vi "test Verify a VI.vi"(8 "error in":errorcluster, 11 "Test Case In":refnum<class "LUnit Extensions Tests.lvclass">) -> (0 "error out":errorcluster, 3 "Test Case Out":refnum<class "LUnit Extensions Tests.lvclass">)   [LabVIEW 2020, in "LUnit Extensions Tests.lvclass"]
uses:
  LUnit Extensions Tests.lvclass
  C:/Program Files/National Instruments/LabVIEW 2026/vi.lib/Astemes/LUnit/Test Case.lvclass
  Source/Extensions/LUnit.Extension/LUnit.Extension.lvlib
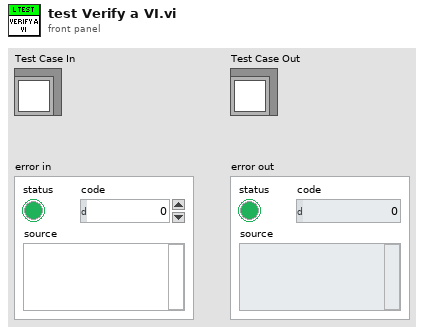
[diagram p1: front panel]
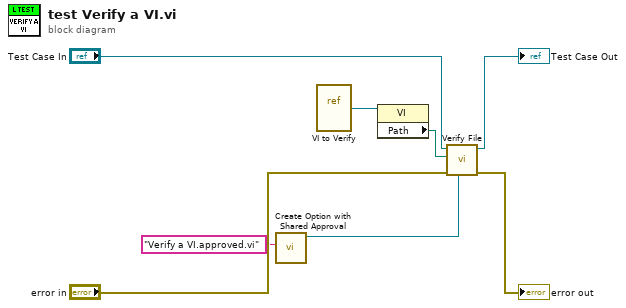
[diagram p0: block diagram]
diagram:
  n1 = call "Create Option with Shared Approval.vi"("Filename"="Verify a VI.approved.vi") -> ("Options outs"=w2:refnum<class "Options.lvclass">)  [unwired: 10 in]
  n2 = vi-ref "VI to Verify.vi"() -> (w4:refnum<vi>)
  n3 = property class="VI"(reference=w4) -> ("Path"=w3:path)  [unwired: 1 in, 2 out]
  n4 = call "Verify File.vi"("Options"=w2, "error in"="error in", "path to file"=w3, "LUnit Test Case In"="Test Case In") -> ("error out"=→"error out":errorcluster, "LUnit Test Case Out"=→"Test Case Out":refnum<class "LUnit Extensions Tests.lvclass">)  [unwired: 6 in]
